vi "valves_pumpprogram.vi"(0 "COM in":refnum<k24>, 1 "Interval (ms)":dbl=15.0 min=1.0 max=100.0, 2 "Timestamp initial":timestamp, 3 "Pump frequency":dbl=15.0 min=1.0 max=100.0, 7 "Pump refnums":T1, 11 "error in (no error)":errorcluster) -> (4 "COM out":refnum<k24>, 6 "Stop?":bool, 15 "error out":errorcluster)   [LabVIEW 2018]
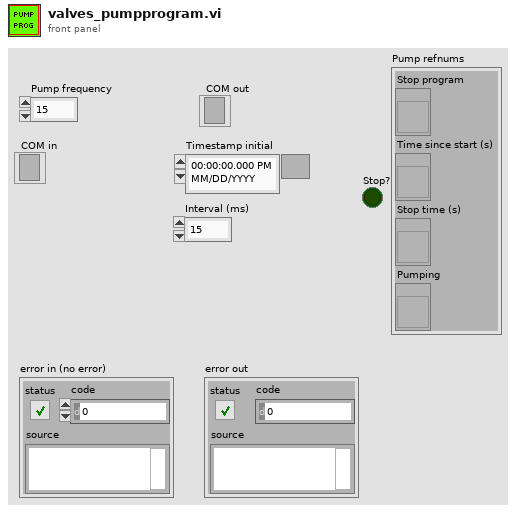
[diagram p1: front panel]
types:
  T1 = cluster{"Stop program":refnum<vi>, "Time since start (s)":refnum<vi>, "Stop time (s)":refnum<vi>, "Pumping":refnum<vi>}
  T2 = cluster{"Step 1":u8[], "Step 2":u8[], "Step 3":u8[], "Step 4":u8[], "Step 5":u8[], "Step 6":u8[]}
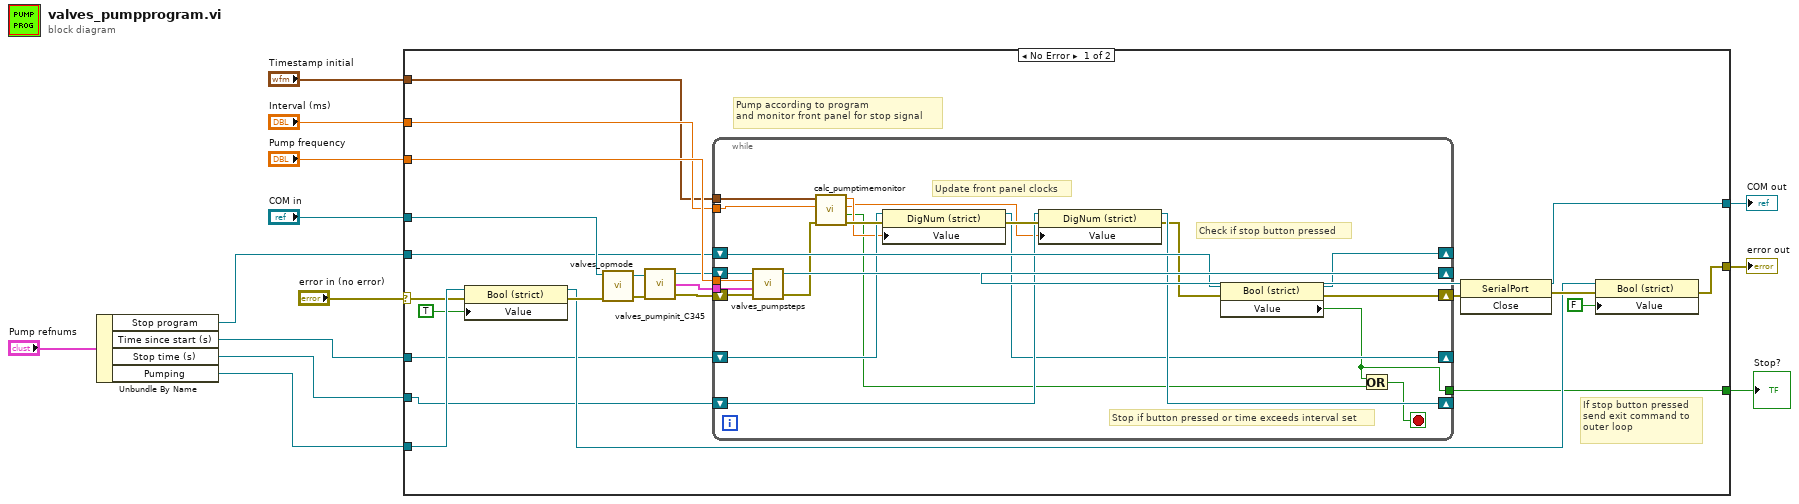
[diagram p0: block diagram]
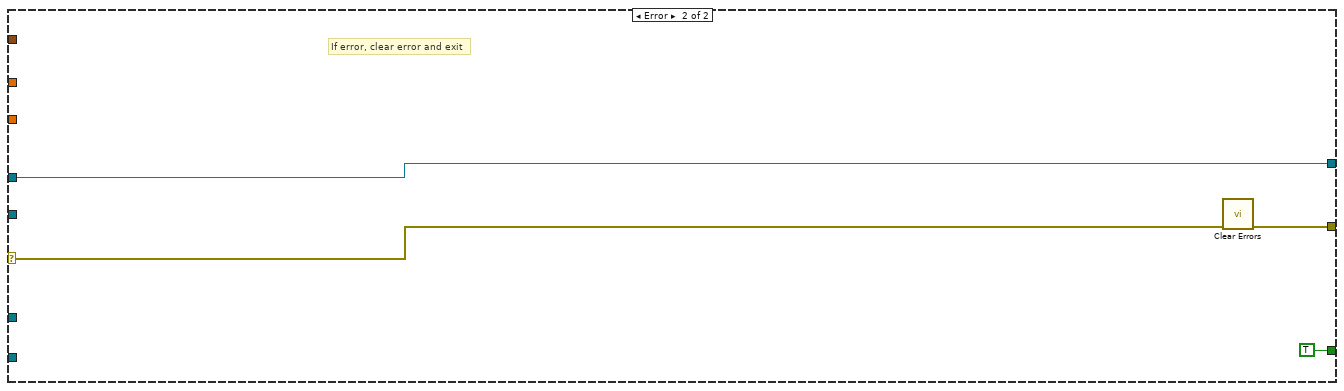
[diagram p2: hidden frame]
diagram:
  n1 = Unbundle By Name("Pump refnums") -> ("Stop program"=w4:refnum<vi>, "Time since start (s)"=w3:refnum<vi>, "Stop time (s)"=w2:refnum<vi>, "Pumping"=w1:refnum<vi>)
  n2 = case shown="No Error" "error in (no error)" {
    selector: "error in (no error)" -> [w17 w63]
    tunnel: [w20 w62] -> w9
    tunnel: "COM in" -> [w37 w64]
    tunnel: [w36 w64] -> w12
    tunnel: "Pump frequency" -> [w35 _]
    tunnel: w4 -> [w21 _]
    tunnel: w1 -> [w25 _]
    tunnel: "Interval (ms)" -> [w19 _]
    tunnel: "Timestamp initial" -> [w18 _]
    tunnel: w3 -> [w16 _]
    tunnel: w2 -> [w15 _]
    tunnel: [w14 TRUE] -> w6
    frame No Error {
      # "If stop button pressed\nsend exit command to\nouter loop"
      # "Pump according to program\nand monitor front panel for stop signal"
      n3 = property class="Bool (strict)"(reference=w25, error in=w17, "Value"=TRUE) -> (reference out=w23:refnum<vi>, error out=w29:errorcluster)
      n4 = call "valves_opmode.vi"("COM4 in"=w37, "error in"=w29) -> ("COM4 out"=w32:refnum<k24>, "error out"=w34:errorcluster)  [unwired: 5 in]
      n5 = call "valves_pumpinit_C345.vi"("COM4 in"=w32, "error in"=w34) -> ("COM4 out"=w31:refnum<k24>, "Commands out"=w30:T2, "error out"=w33:errorcluster)  [unwired: 3 in]
      n6 = while {
        tunnel: w30 -> [w58]
        shift-right: [w57] -> w26
        shift-left: w31 -> [w59]
        tunnel: w35 -> [w56]
        shift-right: [w55] -> w28
        shift-left: w33 -> [w60]
        shift-right: [w53] -> _
        shift-left: w21 -> [w54]
        tunnel: w18 -> [w51]
        tunnel: w19 -> [w50]
        shift-right: [w43] -> _
        shift-left: w15 -> [w46]
        shift-right: [w42] -> _
        shift-left: w16 -> [w47]
        tunnel: [w38] -> w14
        stop <- w39 stop-if-true
        # "Stop if button pressed or time exceeds interval set"
        # "Check if stop button pressed"
        # "Update front panel clocks"
        n7 = call "valves_pumpsteps.vi"("COM4 in"=w59, "Pump frequency"=w56, "Commands in"=w58, "error in"=w60) -> ("COM4 out"=w57:refnum<k24>, "error out"=w52:errorcluster)  [unwired: 3 in]
        n8 = call "calc_pumptimemonitor.vi"("error in (no error)"=w52, "Interval (ms)"=w50, "Initial timestamp"=w51) -> ("error out"=w49:errorcluster, "Stop?"=w40:bool, "Stop time (s)"=w44:dbl, "Time since start (s)"=w45:dbl)  [unwired: 5 in]
        n9 = property class="DigNum (strict)"(reference=w47, error in=w49, "Value"=w45) -> (reference out=w42:refnum<vi>, error out=w48:errorcluster)
        n10 = property class="DigNum (strict)"(reference=w46, error in=w48, "Value"=w44) -> (reference out=w43:refnum<vi>, error out=w41:errorcluster)
        n11 = property class="Bool (strict)"(reference=w54, error in=w41) -> (reference out=w53:refnum<vi>, error out=w55:errorcluster, "Value"=w38:bool)
        n12 = Or(x=w38, y=w40) -> (x .or. y?=w39:bool)
      }
      n13 = invoke class="SerialPort" method="Close"(reference=w26, error in=w28) -> (reference out=w36:refnum<k24>, error out=w27:errorcluster)  [unwired: 1 in, 1 out]
      n14 = property class="Bool (strict)"(reference=w23, error in=w27, "Value"=FALSE) -> (error out=w20:errorcluster)  [unwired: 1 out]
    }
    frame Error {
      # "If error, clear error and exit"
      n15 = call <vilib>:"Clear Errors.vi"("error in (no error)"=w63) -> ("error out"=w62:errorcluster)  [unwired: 5 in, 1 out]
    }
  }
  "error out" <- w9
  "COM out" <- w12
  "Stop?" <- w6
